vi "2.Serrure_Numerique_GJE.vi"() -> ()   [LabVIEW 2018]
panel:
  out "Led":bool
  in  "Button 3":i8(knob) scale=0.0..9.0
  in  "Button 2":i8(knob) scale=0.0..9.0
  in  "Button":i8(knob) scale=0.0..9.0
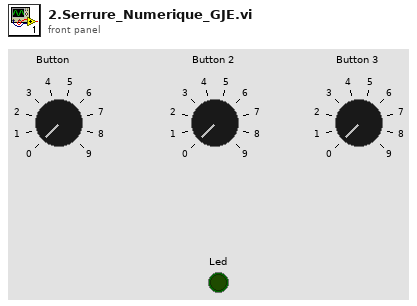
[diagram p1: front panel]
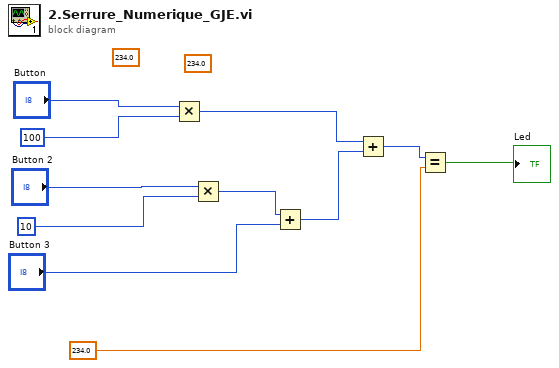
[diagram p0: block diagram]
diagram:
  (unwired) 234.0 ("Button 3")
  (unwired) 234.0 ("Button 2")
  n1 = Multiply(x="Button", y=100) -> (x*y=w7:i32)
  n2 = Multiply(x="Button 2", y=10) -> (x*y=w5:i32)
  n3 = Add(x=w5, y="Button 3") -> (x+y=w1:i32)
  n4 = Add(x=w7, y=w1) -> (x+y=w3:i32)
  n5 = Equal?(x=w3, y=234.0 ("Button")) -> (x = y?=→"Led":bool)
